vi "Helper Action.vi"(8 "error in (no error)":errorcluster, 9 "Message Data":variant, 10 "Message":string, 11 "Mock Process In":refnum<class "Mock Process.lvclass">) -> (0 "error out":errorcluster, 1 "Exit?":bool, 2 "Loop Period [ms]":u32=1000, 3 "Mock Process Out":refnum<class "Mock Process.lvclass">)   [LabVIEW 2020, in "Mock Process.lvclass"]
uses:
  Mock Process.lvclass
  Mock Process.lvclass/Mock Process.ctl
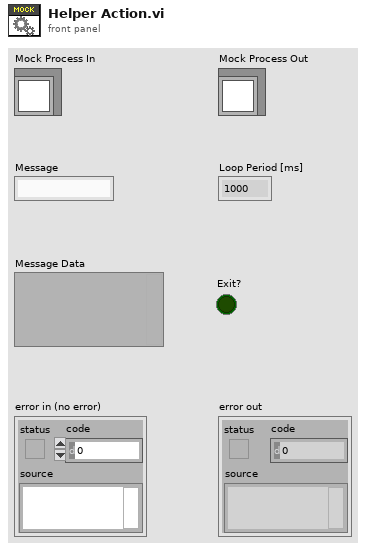
[diagram p1: front panel]
types:
  T1 = cluster{"Message":string, "Message Data":variant}
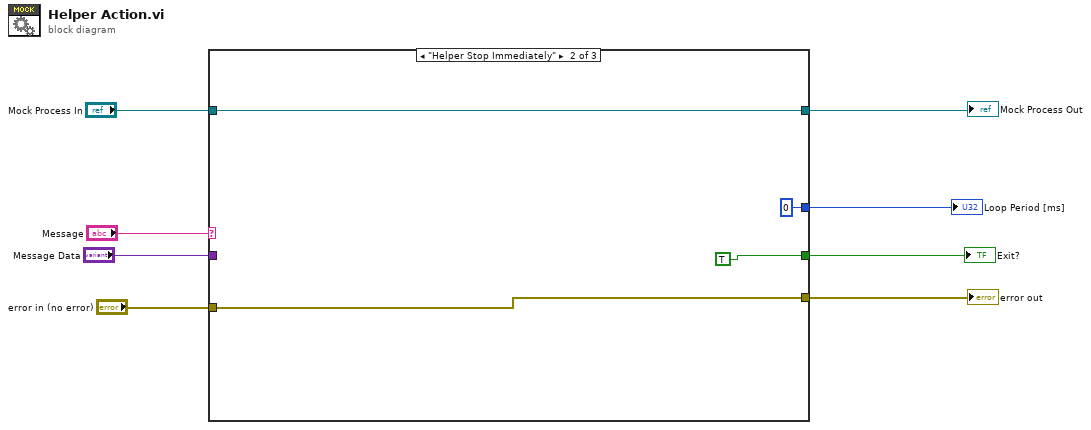
[diagram p0: block diagram]
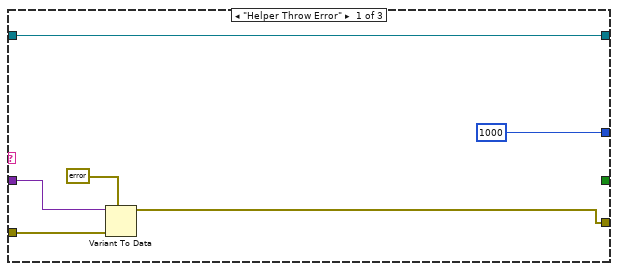
[diagram p2: hidden frame]
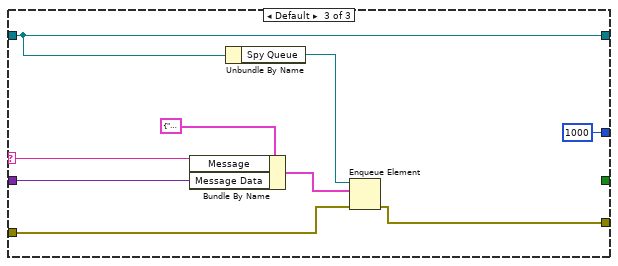
[diagram p3: hidden frame]
diagram:
  n1 = case shown="\"Helper Stop Immediately\"" "Message" {
    selector: "Message" -> [_ _ w24]
    tunnel: "Mock Process In" -> [w10 w18 w22]
    tunnel: [w12 w16 w26] -> w7
    tunnel: "error in (no error)" -> [w13 w16 w25]
    tunnel: "Message Data" -> [w14 _ w23]
    tunnel: [w10 w18 w22] -> w3
    tunnel: [_ TRUE _] -> w2
    tunnel: [u32 1000 ("Loop Period [ms]") u32 0 ("Loop Period [ms]") u32 1000 ("Loop Period [ms]")] -> w1
    frame "Helper Throw Error" {
      n2 = Variant To Data(error in=w13, type=errorcluster {"status"=FALSE, "code"=0, "source"=""} ("error out"), Variant=w14) -> (data=w12:errorcluster)  [unwired: 1 out]
    }
    frame "Helper Stop Immediately" {
    }
    frame Default {
      n3 = Bundle By Name(cluster=T1 {"Message"="", "Message Data"=variant} ("Message Cluster"), "Message"=w24, "Message Data"=w23) -> (w21:T1)
      n4 = Unbundle By Name(w22) -> ("Spy Queue"=w27:refnum<queue>)
      n5 = Enqueue Element(queue=w27, element=w21, error in (no error)=w25) -> (error out=w26:errorcluster)  [unwired: 1 in, 2 out]
    }
  }
  "error out" <- w7
  "Mock Process Out" <- w3
  "Loop Period [ms]" <- w1
  "Exit?" <- w2
